vi "Saturation_Powers.vi"(10 "Right_Motor":dbl, 11 "Left_Motor":dbl) -> (2 "Right_Motor_Say":dbl, 3 "Left_Motor_Sat":dbl)   [LabVIEW 2017, in "ArgosLib.lvlib"]
uses:
  ArgosLib.lvlib
panel:
  # "Saturation_Power"
  # "This subsystem saturates the the motor values and applies extra power to the opposite motor.  This is done to allow for constant turning ratios independent of speed"
  # "Inputs"
  # "Outputs"
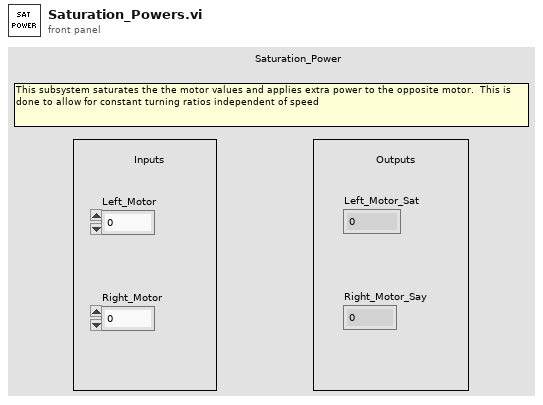
[diagram p1: front panel]
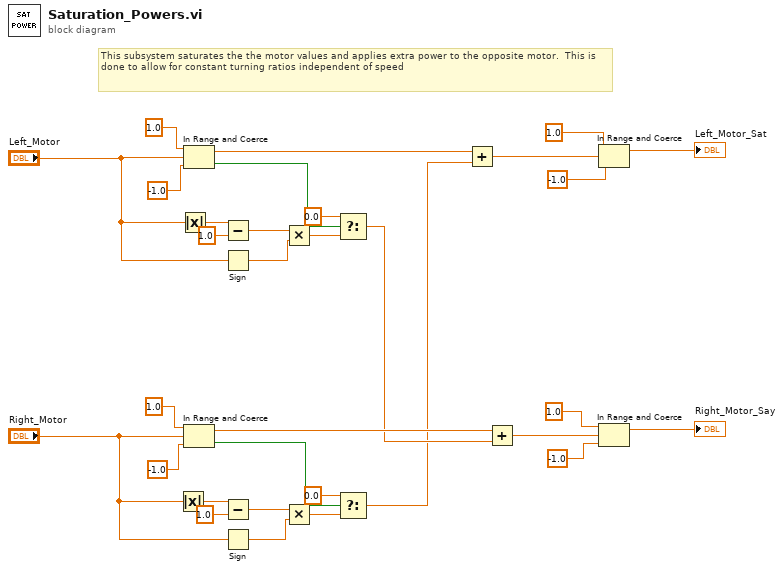
[diagram p0: block diagram]
diagram:
  # "This subsystem saturates the the motor values and applies extra power to the opposite motor.  This is done to allow for constant turning ratios independent of speed"
  n1 = Absolute Value(x="Right_Motor") -> (abs(x)=w20:dbl)
  n2 = Absolute Value(x="Left_Motor") -> (abs(x)=w25:dbl)
  n3 = In Range and Coerce(upper limit=1.0, x="Left_Motor", lower limit=-1.0) -> (coerced(x)=w12:dbl, In Range?=w31:bool)
  n4 = In Range and Coerce(upper limit=1.0, x="Right_Motor", lower limit=-1.0) -> (coerced(x)=w11:dbl, In Range?=w15:bool)
  n5 = Subtract(x=w25, y=1.0) -> (x-y=w28:dbl)
  n6 = Sign(1:"Left_Motor") -> (0:w29:dbl)
  n7 = Subtract(x=w20, y=1.0) -> (x-y=w18:dbl)
  n8 = Sign(1:"Right_Motor") -> (0:w17:dbl)
  n9 = Multiply(x=w28, y=w29) -> (x*y=w30:dbl)
  n10 = Multiply(x=w18, y=w17) -> (x*y=w16:dbl)
  n11 = Select(t=0.0, s=w31, f=w30) -> (s? t:f=w10:dbl)
  n12 = Select(t=0.0, s=w15, f=w16) -> (s? t:f=w9:dbl)
  n13 = Add(x=w12, y=w9) -> (x+y=w8:dbl)
  n14 = Add(x=w11, y=w10) -> (x+y=w2:dbl)
  n15 = In Range and Coerce(upper limit=1.0, x=w8, lower limit=-1.0) -> (coerced(x)=→"Left_Motor_Sat":dbl)  [unwired: 1 out]
  n16 = In Range and Coerce(upper limit=1.0, x=w2, lower limit=-1.0) -> (coerced(x)=→"Right_Motor_Say":dbl)  [unwired: 1 out]
